vi "HL Grab.vi"() -> ()   [LabVIEW 2017]
doc: "The HL Grab VI acquires images continuously and displays the images in an image control using high-level acquisition VIs. A grab is appropriate for high-speed applications that process only one image at a time."
uses:
  <vilib>/Analysis/NI_AALBase.lvlib
panel:
  out "mean pixel value":u16
  out "Acquisition Rate (Hz)":dbl
  out "Histogram Graph":T1(graph)
  out "Display Rate (Hz)":dbl
  out "Image":T2(plugin-control)
  in  "Interface Name":string="img0"
  in  "Stop":bool
  # "Overview: Demonstrates how to perform acquires images continuously and displays the images in an image control using high-level acquisition VIs. \nRequirements: Vision Acquisition Software, IMAQ frame grabber.\nInstructions: \n1. Select the IMAQ frame grabber Interface Name.\n2. Run the VI."
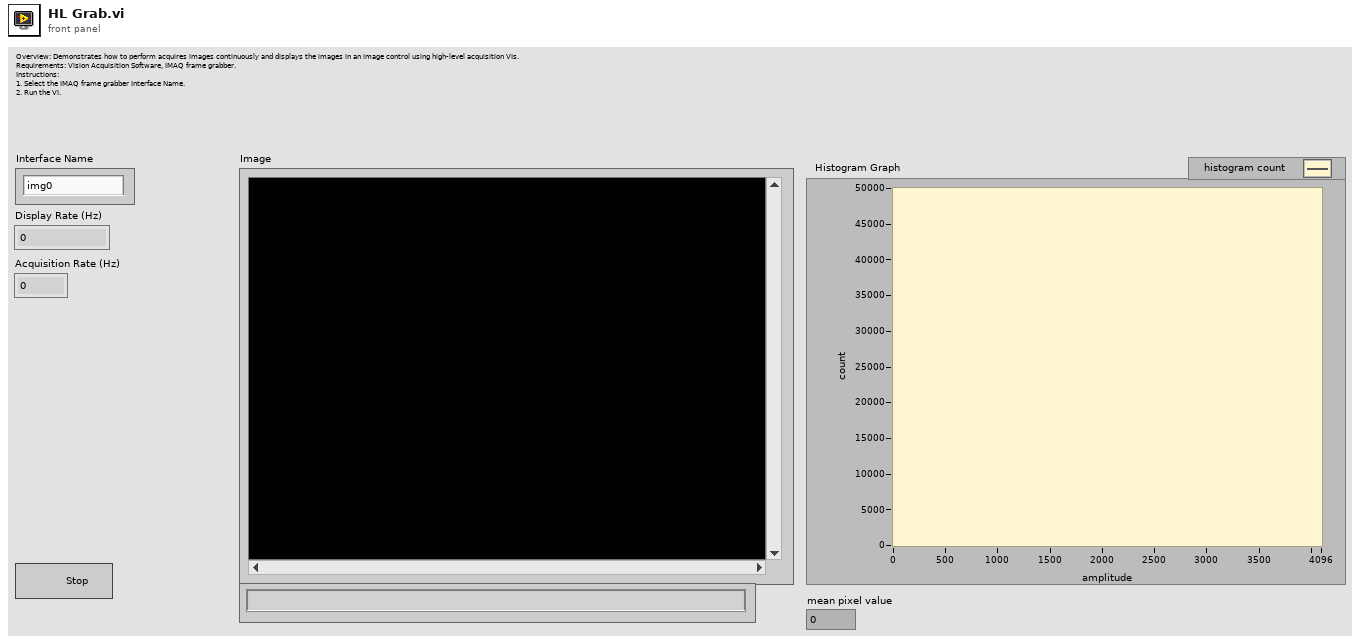
[diagram p1: front panel]
types:
  T1 = cluster{"X Values":dbl[], "Histogram: h(x)":i32[]}
  T2 = typedef "IMAQ Image.ctl" = refnum<image>
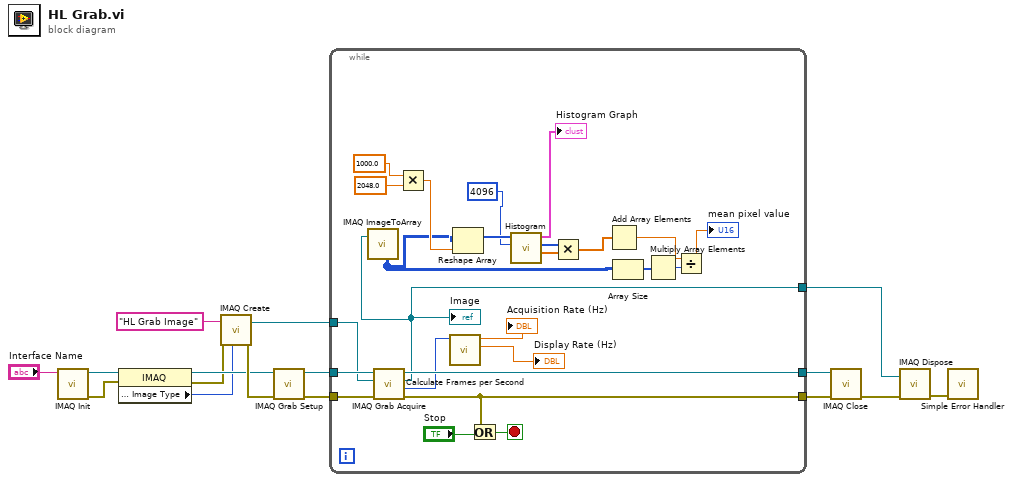
[diagram p0: block diagram]
diagram:
  n1 = call <vilib>:"IMAQ Init.vi"("Interface Name"="Interface Name") -> ("error out"=w8:errorcluster, "IMAQ Session Out"=w9:refnum<k11>)  [unwired: 1 in, 8 out]
  n2 = property class="IMAQ"(reference=w9, error in=w8) -> (reference out=w7:refnum<k11>, error out=w6:errorcluster, "Image Parameters : Image Type"=w5:u32)
  n3 = call "IMAQ Create"("Image Name"="HL Grab Image", "Image Type"=w5, "error in (no error)"=w6) -> ("New Image"=w15:T2, "error out"=w16:errorcluster)  [unwired: 1 in, 1 out]
  n4 = call <vilib>:"IMAQ Grab Setup.vi"("error in (no error)"=w16, "IMAQ Session In"=w7) -> ("error out"=w13:errorcluster, "IMAQ Session Out"=w14:refnum<k11>)  [unwired: 8 out]
  n5 = while {
    tunnel: [w36] -> w10
    tunnel: w15 -> [w39]
    tunnel: w14 -> [w40]
    tunnel: w13 -> [w41]
    tunnel: [w35] -> w4
    tunnel: [w32] -> w2
    stop <- w38 stop-if-true
    n6 = call <vilib>:"IMAQ Grab Acquire.vi"("error in (no error)"=w41, "Image In"=w39, "IMAQ Session In"=w40) -> ("error out"=w35:errorcluster, "Acquired Buffer Number"=w34:u32, "Image Out"=w32:T2, "IMAQ Session Out"=w36:refnum<k11>)  [unwired: 1 in, 4 out]
    "Image" <- w32
    n7 = call "IMAQ ImageToArray"("Image"=w32) -> ("Image Pixels (U16)"=w21:u16[][])  [unwired: 3 in, 4 out]
    n8 = Multiply(x=1000.0, y=2048.0) -> (x*y=w26:dbl)
    n9 = call <vilib>:"Calculate Frames per Second.vi"("Buffer Number"=w34) -> ("Processed Frames/s"=→"Display Rate (Hz)":dbl, "Acquired Frames/s"=→"Acquisition Rate (Hz)":dbl)  [unwired: 8 in, 1 out]
    n10 = Reshape Array(w21, w26) -> (w31:u16[])
    n11 = Or(x=w35, y="Stop") -> (x .or. y?=w38:bool)
    n12 = call <vilib>:"Histogram.vi"("intervals"=4096 ("samples"), "X"=w31) -> ("X Values"=w24:dbl[], "Histogram: h(x)"=w23:i32[], "Histogram Graph"=→"Histogram Graph":T1)  [unwired: 6 in, 1 out]
    n13 = Multiply(x=w23, y=w24) -> (x*y=w22:dbl[])
    n14 = Add Array Elements(numeric array=w22) -> (sum=w20:dbl)
    n15 = Array Size(array=w21) -> (size(s)=w18:i32[])
    n16 = Multiply Array Elements(1:w18) -> (0:w17:i32)
    n17 = Divide(x=w20, y=w17) -> (x/y=→"mean pixel value":dbl)
  }
  n18 = call <vilib>:"IMAQ Close.vi"("error in (no error)"=w4, "IMAQ Session In"=w10) -> ("error out"=w3:errorcluster)  [unwired: 9 out]
  n19 = call "IMAQ Dispose"("Image"=w2, "error in (no error)"=w3) -> ("error out"=w1:errorcluster)  [unwired: 1 in, 3 out]
  n20 = call <vilib>:"Simple Error Handler.vi"("error in (no error)"=w1) -> ()  [unwired: 1 in, 8 out]
